vi "LFU Get File Size__ogtk.vi"(4 "error in (no error)":errorcluster, 7 "handle":u32) -> (0 "error out":errorcluster, 1 "file size":dbl, 3 "handle out":u32)   [LabVIEW 2020]
doc: "Low level utility function to retrieve the size of a file as double precision number to work for files larger than 2GB."
uses:
  kernel32.dll
panel:
  # "LFU Get File Size.vi\n\nPlease visit http://www.OpenG.org to learn about the\nOpen Source LabVIEW software movement.\n\nNOTICE -- YOU MUST LEAVE THIS NOTICE IN PLACE.  PER THE TERMS OF THE LICENSE BELOW, YOU MAY SUBLICENSE THIS SOFTWARE \nIN ANY WAY THAT DOES NOT CONFLICT WITH THIS LICENSE.\n\n### BSD License (http://www.opensource.org/licenses/bsd-license.php) Begin ###\n\nCopyright (c) 2003, Rolf Kalbermatter <rolf.kalbermatter@citeng.com>\n\nAll rights reserved.\n\nRedistribution and use in source and binary forms, with or without modification, are permitted provided that the following conditions are met:\n\n    * Redistributions of source code must retain the above copyright notice, this list of conditions and the following disclaimer.\n    * Redistributions in binary form must reproduce the above copyright notice, this list of conditions and the following disclaimer in the \n       documentation and/or other materials provided with the distribution.\n    * Neither the name of SciWare, James Kring, Inc., nor the names of its contributors may be used to endorse or promote products derived \n       from this software without specific prior written permission.\n\nTHIS SOFTWARE IS PROVIDED BY THE COPYRIGHT HOLDERS AND CONTRIBUTORS \"AS IS\" AND ANY EXPRESS OR IMPLIED WARRANTIES, \nINCLUDING, BUT NOT LIMITED TO, THE IMPLIED WARRANTIES OF MERCHANTABILITY AND FITNESS FOR A PARTICULAR PURPOSE ARE \nDISCLAIMED. IN NO EVENT SHALL THE COPYRIGHT OWNER OR CONTRIBUTORS BE LIABLE FOR ANY DIRECT, INDIRECT, INCIDENTAL,\n SPECIAL, EXEMPLARY, OR CONSEQUENTIAL DAMAGES (INCLUDING, BUT NOT LIMITED TO, PROCUREMENT OF SUBSTITUTE GOODS OR \nSERVICES; LOSS OF USE, DATA, OR PROFITS; OR BUSINESS INTERRUPTION) HOWEVER CAUSED AND ON ANY THEORY OF LIABILITY, \nWHETHER IN CONTRACT, STRICT LIABILITY, OR TORT (INCLUDING NEGLIGENCE OR OTHERWISE) ARISING IN ANY WAY OUT OF THE USE \nOF THIS SOFTWARE, EVEN IF ADVISED OF THE POSSIBILITY OF SUCH DAMAGE.\n\n### BSD License End ###"
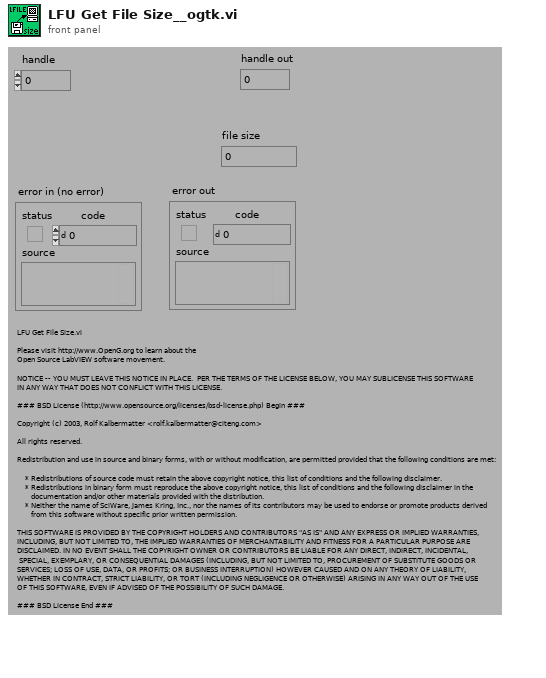
[diagram p1: front panel]
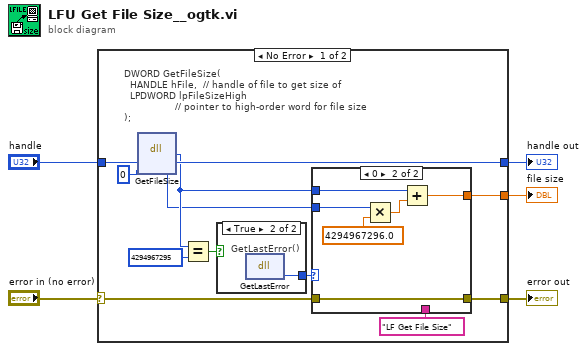
[diagram p0: block diagram]
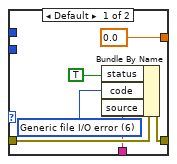
[diagram p2: hidden frame]
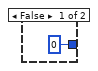
[diagram p3: hidden frame]
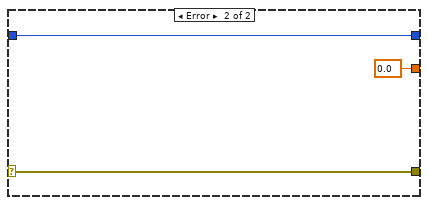
[diagram p4: hidden frame]
diagram:
  n1 = case shown="No Error" "error in (no error)" {
    selector: "error in (no error)" -> [w8 w33]
    tunnel: [w17 w34] -> w5
    tunnel: "handle" -> [w16 w34]
    tunnel: [w7 w33] -> w2
    tunnel: [w6 0.0] -> w1
    frame No Error {
      # "DWORD GetFileSize(\n  HANDLE hFile,  // handle of file to get size of\n  LPDWORD lpFileSizeHigh \n                 // pointer to high-order word for file size\n);"
      n2 = dll-call lib="kernel32.dll" fn="GetFileSize"("handle"=w16, "sizeHigh"=0 ("overlapped")) -> (w10:u32, "handle"=w17:u32, "sizeHigh"=w9:i32)  [unwired: 3 in, 2 out]
      n3 = Equal?(x=w10, y=u32 4294967295) -> (x = y?=w13:bool)
      n4 = case shown="True" w13 {
        tunnel: [u32 0 w31] -> w11
        frame False {
        }
        frame True {
          # "GetLastError()"
          n5 = dll-call lib="kernel32.dll" fn="GetLastError"() -> (w31:u32)  [unwired: 3 in, 2 out]
        }
      }
      n6 = case shown="0" w11 {
        tunnel: w9 -> [_ w29]
        tunnel: [0.0 w26] -> w6
        tunnel: w10 -> [_ w25]
        tunnel: w8 -> [w22 w24]
        tunnel: [w21 w24] -> w7
        tunnel: "LF Get File Size" ("source") -> [w18 _]
        frame Default {
          w19 = 6 items=["No error", "Argument error", "Memory is full", "Out of zone", "End of file", "File already open", "Generic file I/O error", "File not found", "File permission error", "Disk is full", "Duplicate path", "Too many files open", "System feature not enabled", "Resource file not found", "Cannot add resource", "Resource not found", "Image not found", "Image memory error", "Pen does not exist", "Config type invalid", "Config token not found", "Config parse error", "Config memory error", "Bad external code format", "Bad external code offset", "External code not present", "Null window", "Destroy window error", "Null menu", "Print aborted", "Bad print record", "Print driver error", "Windows error during printing", "Memory error during printing", "Print dialog error", "Generic print error", "Invalid device refnum", "Device not found", "Device parameter error", "Device unit error", "Cannot open device", "Device call aborted", "Generic error", "Cancelled by user", "Object ID too low", "Object ID too high", "Object not in heap", "Unknown heap", "Unknown object (invalid DefProc)", "Unknown object (DefProc not in table)", "Message out of range", "Invalid (null) method", "Unknown message", "Manager call not supported", "Bad address", "Network operation in progress", "Network operation timed out", "Connection is busy", "Network attribute not supported", "Network error", "Address in use", "System out of memory", "Connection aborted", "Connection refused", "Not connected", "Already connected", "Connection closed", "Initialization error (interapplication manager)", "Bad occurrence", "Wait on unbound occurrence handler", "Occurrence queue overflow", "Datalog type conflict", "Unused", "Unrecognized type (interapplication manager)", "Memory corrupt", "Failed to make temporary DLL", "Old CIN version", "Drag socket not found", "Failed to load drop-object", "Failed to register OLE object", "Failed to release OLE object", "Format specifier type mismatch", "Unknown format specifier", "Too few format specifiers", "Too many format specifiers", "Scan failed", "Newer CIN version", "Error converting to variant", "Runtime menu error", "Password tampered", "Variant attribute not found", "Incompatible variant data type", "Event data is not available", "Event Store is not present", "Occurrence is not found", "Event Queue is not created", "Event info is not available", "Refnum passed is NULL", "Error retrieving Class GUID", "Error retrieving CoClass GUID", "Error retrieving TypeLib GUID.", "Bad built application magic bytes.", "Specific driver is different from the specific driver associated with the Logical Name.", "There is no session opened to the class driver.", "Max Error", "MAX - Error with config objects", "MAX - Error loading configuration", "MAX - Group not supported"]
          n7 = Bundle By Name(cluster=w22, "status"=TRUE, "code"=w19, "source"=w18) -> (w21:errorcluster)
        }
        frame 0 {
          n8 = Multiply(x=w29, y=4294967296.0) -> (x*y=w27:dbl)
          n9 = Add(x=w25, y=w27) -> (x+y=w26:dbl)
        }
      }
    }
    frame Error {
    }
  }
  "handle out" <- w5
  "error out" <- w2
  "file size" <- w1
